vi "numberInputOutput1.vi"() -> ()   [LabVIEW 2021]
panel:
  in  "Knob":dbl(knob) scale=0.0..10.0
  out "Gauge":dbl(knob) scale=0.0..10.0
  out "Meter":dbl(knob) scale=0.0..100.0
  out "Output":dbl
  in  "Input":dbl
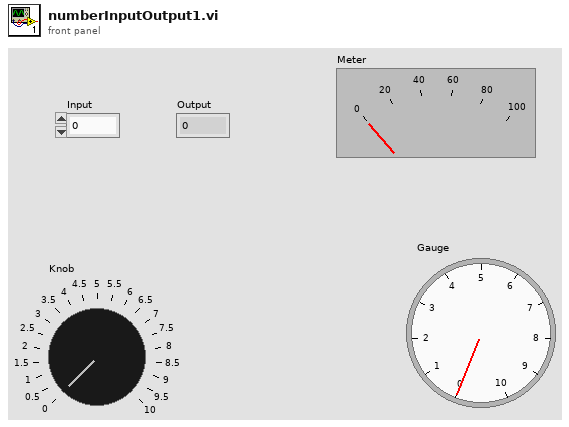
[diagram p1: front panel]
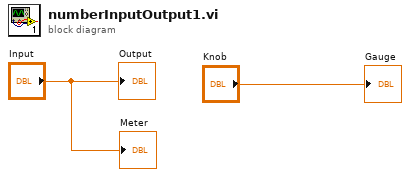
[diagram p0: block diagram]
diagram:
  "Output" <- "Input"
  "Meter" <- "Input"
  "Gauge" <- "Knob"
